vi "area.vi"(10 "height":i32, 11 "width":i32) -> (3 "function return":i32)   [LabVIEW 2013, in "OpencvLabviewTest.lvlib"]
doc: "__declspec(dllexport) int area(int width, int height)\n\n__declspec(dllexport) int area(int width, int height);"
uses:
  OpencvLabviewTest.lvlib
  OpencvLabviewTest.dll
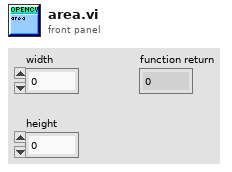
[diagram p1: front panel]
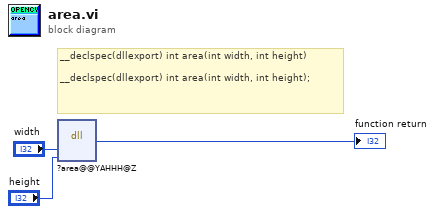
[diagram p0: block diagram]
diagram:
  # "__declspec(dllexport) int area(int width, int height)\n\n__declspec(dllexport) int area(int width, int height);"
  n1 = dll-call lib="D:/congxin/labview/OpencvLabviewTest/subvi/OpencvLabviewTest.*" fn="?area@@YAHHH@Z"("width"="width", "height"="height") -> (→"function return":i32)  [unwired: 5 in, 2 out]
